vi "GetVariableValues.vi"(8 "error in (no error)":errorcluster, 10 "SequenceStep":i32, 11 "VariablesManager in":refnum<class "VariableManager.lvclass">) -> (0 "error out":errorcluster, 2 "VariableValues":refnum<class "VariableValue.lvclass">[](array[class]), 3 "VariablesManager out":refnum<class "VariableManager.lvclass">)   [LabVIEW 2013, in "VariableManager.lvclass"]
doc: "Return variable values at the given sequence step, if SequenceStep is in the range [0, MaxSteps-1] \nReturn default variable values, if SequenceStepIn is outside the range [0, MaxSteps-1]\n\nAn error is thrown if a sequence function cannot be evaluated."
uses:
  VariableManager.lvclass
  VariableValue/VariableValue.lvclass
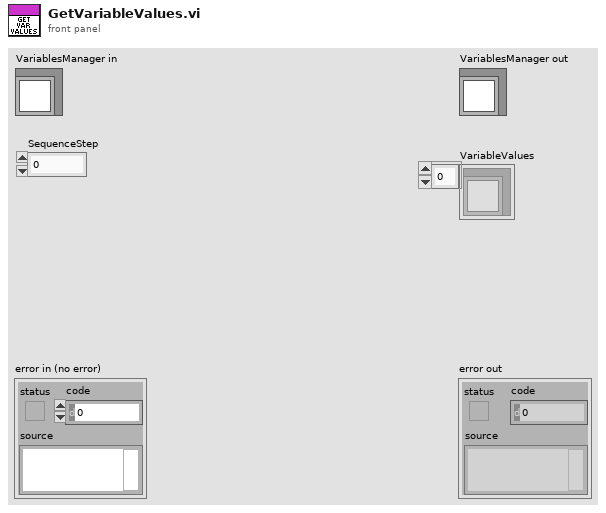
[diagram p1: front panel]
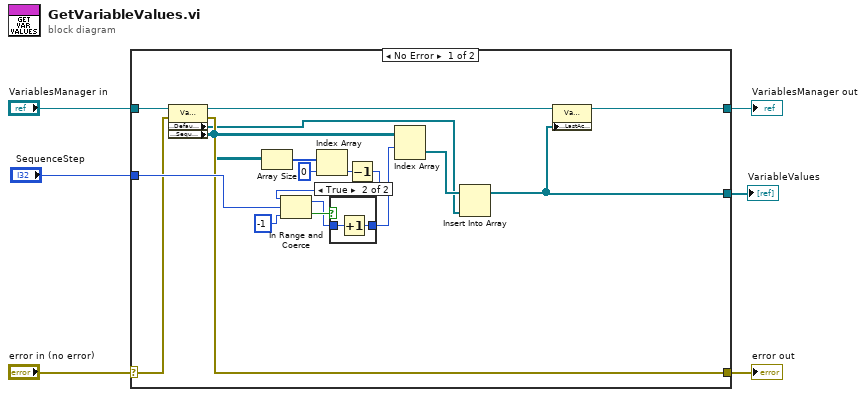
[diagram p0: block diagram]
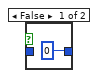
[diagram p2: hidden frame]
diagram:
  n1 = case shown="No Error" "error in (no error)" {
    selector: "error in (no error)" -> [w10 w29]
    tunnel: [w11 w29] -> w5
    tunnel: [w14 w28] -> w3
    tunnel: "VariablesManager in" -> [w12 w28]
    tunnel: "SequenceStep" -> [w19 _]
    tunnel: [w9 _] -> w1
    frame No Error {
      n2 = property class="VariableManager.lvclass"(reference=w12, error in=w10) -> (reference out=w15:refnum<class "VariableManager.lvclass">, error out=w11:errorcluster, "Accessors:DefaultValues"=w7:refnum<class "VariableValue.lvclass">[], "Accessors:SequenceValues"=w8:refnum<class "VariableValue.lvclass">[][])
      n3 = Array Size(array=w8) -> (size(s)=w24:i32[])
      n4 = Index Array(array=w24, index=0) -> (element=w22:i32)
      n5 = Decrement(x=w22) -> (x-1=w21:i32)
      n6 = In Range and Coerce(upper limit=w21, x=w19, lower limit=-1) -> (coerced(x)=w17:i32, In Range?=w18:bool)
      n7 = case shown="True" w18 {
        tunnel: w17 -> [_ w27]
        tunnel: [0 ("lower limit") w26] -> w16
        frame False {
        }
        frame True {
          n8 = Increment(x=w27) -> (x+1=w26:i32)
        }
      }
      n9 = Index Array(array=w8, index (row)=w16) -> (element=w13:refnum<class "VariableValue.lvclass">[])  [unwired: 1 in]
      n10 = Insert Into Array(array=w13, new element=w7) -> (w9:refnum<class "VariableValue.lvclass">[])  [unwired: 1 in]
      n11 = property class="VariableManager.lvclass"(reference=w15, "Accessors:LastAcquireValues"=w9) -> (reference out=w14:refnum<class "VariableManager.lvclass">)  [unwired: 1 in, 1 out]
    }
    frame Error {
    }
  }
  "error out" <- w5
  "VariablesManager out" <- w3
  "VariableValues" <- w1
